vi "Create Client.vi"(8 "error in":errorcluster, 11 "cluster id":string) -> (0 "error out":errorcluster, 3 "grpc client id":T1)   [LabVIEW 2020, in "Measurement Plugin Session Management V1.lvlib" / "Session Reservation.lvclass"]
uses:
  Session Reservation.lvclass
  <vilib>/gRPC/LabVIEW gRPC Library/Shared/grpcId.ctl
  gRPC/Generated APIs/ni/measurementlink/discovery/v1/RPC Messages/ni_measurementlink_discovery_v1_ResolveServiceRequest.ctl
  gRPC/Generated APIs/ni/measurementlink/sessionmanagement/v1/ni.measurementlink.sessionmanagement.v1.lvlib
  Measurement Plugin Discovery V1/Measurement Plugin Discovery V1.lvlib
  gRPC/Generated APIs/ni/measurementlink/discovery/v1/ni.measurementlink.discovery.v1.lvlib
  <vilib>/gRPC/LabVIEW gRPC Library/grpc-lvsupport-release.lvlib
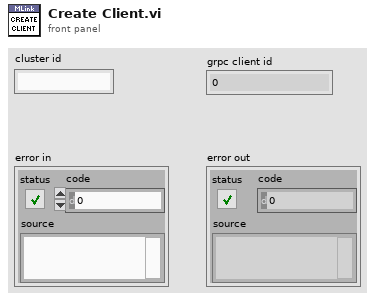
[diagram p1: front panel]
types:
  T1 = typedef "grpc-lvsupport-release.lvlib/grpcId.ctl" = u64
  T2 = typedef "ni.measurementlink.discovery.v1.lvlib/ni_measurementlink_discovery_v1_ResolveServiceRequest.ctl" = cluster{"provided_interface":string, "service_class":string}
  T3 = typedef "ni.measurementlink.discovery.v1.lvlib/ni_measurementlink_discovery_v1_ServiceLocation.ctl" = cluster{"location":string, "insecure_port":string, "ssl_authenticated_port":string}
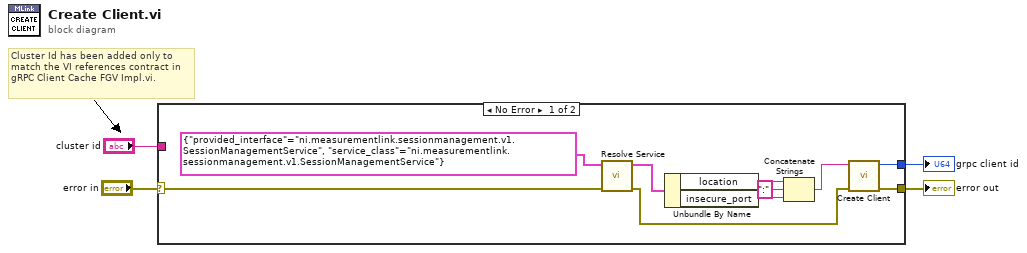
[diagram p0: block diagram]
diagram:
  # "Cluster Id has been added only to match the VI references contract in gRPC Client Cache FGV Impl.vi."
  n1 = case shown="No Error" "error in" {
    selector: "error in" -> [w12 w15]
    tunnel: [w11 _] -> w3
    tunnel: [w10 w15] -> w2
    tunnel: "cluster id" -> [_ _]
    frame No Error {
      n2 = call "Resolve Service.vi"("error in"=w12, "request data"=T2 {"provided_interface"="ni.measurementlink.sessionmanagement.v1.SessionManagementService", "service_class"="ni.measurementlink.sessionmanagement.v1.SessionManagementService"}) -> ("error out"=w13:errorcluster, "response data"=w14:T3)  [unwired: 8 in]
      n3 = Unbundle By Name(w14) -> ("location"=w6:string, "insecure_port"=w7:string)
      n4 = Concatenate Strings(w6, ":" ("string"), w7) -> (w9:string)
      n5 = call "Create Client.vi"("error in"=w13, "address"=w9) -> ("error out"=w10:errorcluster, "gRPC ID Out"=w11:T1)  [unwired: 8 in]
    }
    frame Error {
    }
  }
  "grpc client id" <- w3
  "error out" <- w2
